vi "test.vi"() -> ()   [LabVIEW 2025]
uses:
  <vilib>/userDefined/High Color/IMAQdx.ctl
  <vilib>/httpClient/POSTBuffer.vi
  <vilib>/vision/driver/NI_Vision_Acquisition_Software.lvlib
  <vilib>/httpClient/LabVIEWHTTPClient.lvlib
  <vilib>/smtpClient/LabVIEWSMTPClient.lvlib
  <vilib>/vision/NI_Vision_Development_Module.lvlib
panel:
  out "Image":T1(plugin-control)
  in  "Salvare imagine":bool
  in  "Pornire achizitie locala imagini":bool
  in  "Stop server":bool
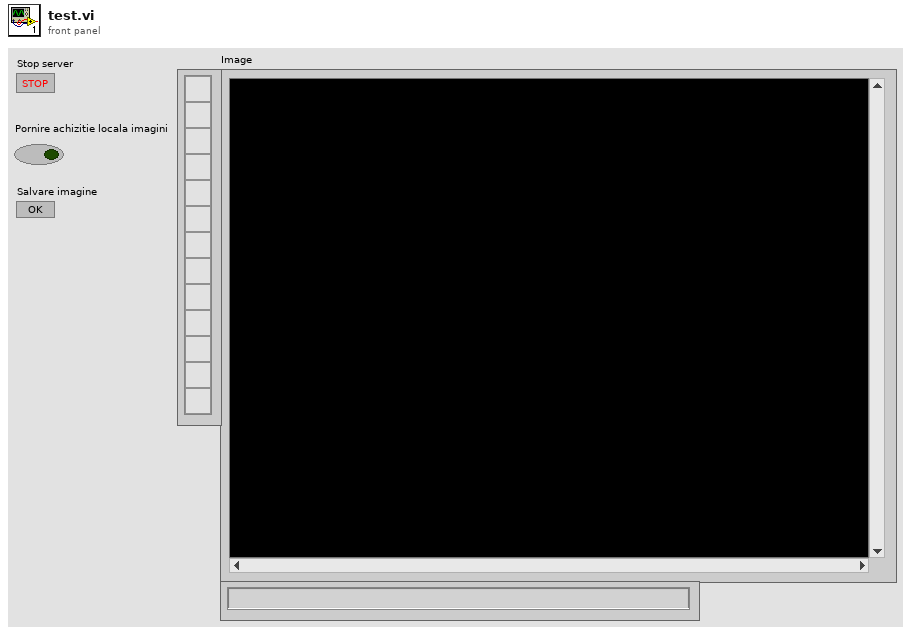
[diagram p1: front panel]
types:
  T1 = typedef "IMAQ Image.ctl" = refnum<image>
  T2 = typedef "Image Type" = u32
  T3 = typedef "IMAQdx.ctl" = refnum<k21>
  T4 = typedef "LabVIEWHTTPClient.lvlib/ClientHandle.ctl" = refnum<k1>
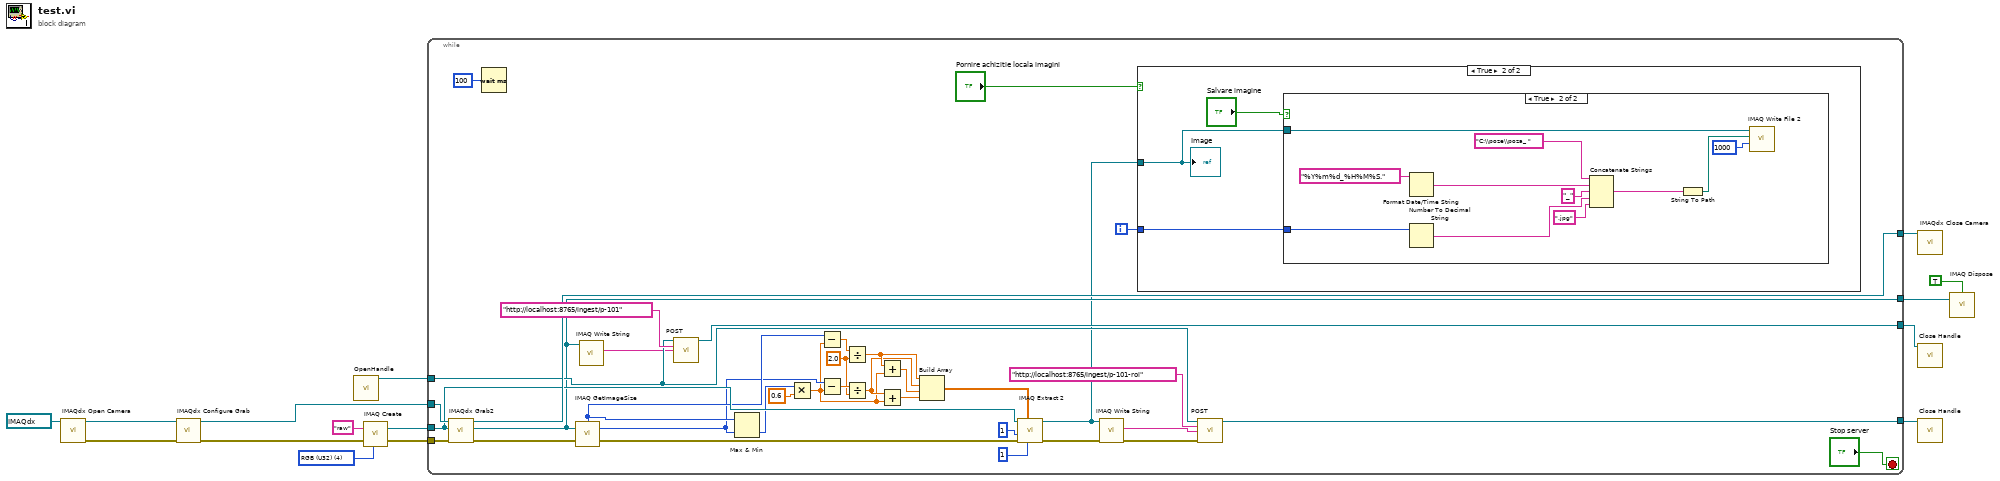
[diagram p0: block diagram]
diagram:
  w3 = T2 4 items=["Grayscale (U8)", "Grayscale (I16)", "Grayscale (SGL)", "Complex (CSG)", "RGB (U32)", "HSL (U32)", "RGB (U64)", "Grayscale (U16)"] ("Image Type")
  n1 = call <vilib>:"IMAQdx Open Camera.vi"("Session In"=T3 "cam1") -> ("error out"=w10:errorcluster, "Session Out"=w13:T3)  [unwired: 9 in]
  n2 = call <vilib>:"IMAQdx Configure Grab.vi"("error in"=w10, "Session In"=w13) -> ("error out"=w9:errorcluster, "Session Out"=w12:T3)  [unwired: 8 in]
  n3 = call <vilib>:"OpenHandle.vi"() -> ("client handle out"=w7:T4)  [unwired: 14 in, 1 out]
  n4 = call "IMAQ Create"("Image Name"="raw", "Image Type"=w3, "error in (no error)"=w9) -> ("New Image"=w14:T1, "error out"=w2:errorcluster)  [unwired: 2 in]
  n5 = while {
    tunnel: w14 -> [w44]
    tunnel: w12 -> [w51]
    tunnel: [w50] -> w11
    tunnel: [w49] -> w8
    tunnel: w7 -> [w45]
    tunnel: [w23] -> w5
    tunnel: w2 -> [w27]
    tunnel: [w30] -> w1
    i -> [w16]
    stop <- "Stop server" stop-if-true
    w37 = 2.0 ("y")
    n6 = call <vilib>:"IMAQdx Grab2.vi"("error in"=w27, "Image In"=w44, "Session In"=w51) -> ("error out"=w26:errorcluster, "Image Out"=w23:T1, "Session Out"=w50:T3)  [unwired: 5 in, 1 out]
    n7 = Wait (ms)(milliseconds to wait=u32 100 ("millisecond timer value")) -> ()  [unwired: 1 out]
    n8 = call "IMAQ GetImageSize"("Image"=w23, "error in (no error)"=w26) -> ("Y Resolution"=w39:i32, "X Resolution"=w43:i32, "error out"=w25:errorcluster)  [unwired: 2 in]
    n9 = call-poly "IMAQ Write String"("Image"=w23) -> ("FileString"=w22:string)  [unwired: 8 in, 2 out]
    n10 = call-poly <vilib>:"POST.vi"("client handle"=w45, "url"="http://localhost:8765/ingest/p-101", "buffer"=w22) -> ("client handle out"=w49:T4)  [unwired: 9 in, 3 out]
    n11 = Max & Min(x=w43, y=w39) -> (min(x,y)=w41:i32)  [unwired: 1 out]
    n12 = Multiply(x=w41, y=0.6) -> (x*y=w33:dbl)
    n13 = Subtract(x=w43, y=w33) -> (x-y=w40:dbl)
    n14 = Subtract(x=w39, y=w33) -> (x-y=w38:dbl)
    n15 = Divide(x=w40, y=w37) -> (x/y=w36:dbl)
    n16 = Divide(x=w38, y=w37) -> (x/y=w34:dbl)
    n17 = Add(x=w36, y=w33) -> (x+y=w35:dbl)
    n18 = Add(x=w34, y=w33) -> (x+y=w32:dbl)
    n19 = Build Array "Build Array"(w36, w34, w35, w32) -> (w31:dbl[])
    n20 = call "IMAQ Extract 2"("Y Step Size"=1, "Optional Rectangle"=w31, "error in (no error)"=w25, "X Step Size"=1, "Image Src"=w44) -> ("error out"=w20:errorcluster, "Image Dst Out"=w17:T1)  [unwired: 5 in]
    n21 = call-poly "IMAQ Write String"("error in (no error)"=w20, "Image"=w17) -> ("error out"=w19:errorcluster, "FileString"=w21:string)  [unwired: 7 in, 1 out]
    n22 = case shown="True" "Pornire achizitie locala imagini" {
      tunnel: w17 -> [_ w52]
      tunnel: w16 -> [_ w53]
      frame False {
      }
      frame True {
        n23 = case shown="True" "Salvare imagine" {
          tunnel: w52 -> [_ w56]
          tunnel: w53 -> [_ w61]
          frame False {
          }
          frame True {
            n24 = Format Date/Time String(time format string (%c)="%Y%m%d_%H%M%S.") -> (date/time string=w63:string)  [unwired: 2 in]
            n25 = Number To Decimal String(number=w61) -> (decimal integer string=w59:string)  [unwired: 1 in]
            n26 = Concatenate Strings "Concatenate Strings"("C:\\poze\\poza_ " ("string"), w63, "_" ("string"), w59, ".jpg" ("string")) -> (w62:string)
            n27 = String To Path(string=w62) -> (path=w57:path)
            n28 = call-poly "IMAQ Write File 2"("Image Quality"=u32 1000, "File Path"=w57, "Image"=w56) -> ()  [unwired: 7 in, 2 out]
          }
        }
        "Image" <- w52
      }
    }
    n29 = call-poly <vilib>:"POST.vi"("client handle"=w45, "url"="http://localhost:8765/ingest/p-101-roi", "buffer"=w21, "error in (no error)"=w19) -> ("client handle out"=w30:T4)  [unwired: 8 in, 3 out]
  }
  n30 = call <vilib>:"IMAQdx Close Camera.vi"("Session In"=w11) -> ()  [unwired: 10 in, 1 out]
  n31 = call <vilib>:"Close Handle.vi"("handle in"=w8) -> ()  [unwired: 13 in, 2 out]
  n32 = call <vilib>:"Close Handle.vi"("handle in"=w1) -> ()  [unwired: 13 in, 2 out]
  n33 = call "IMAQ Dispose"("All Images? (No)"=TRUE, "Image"=w5) -> ()  [unwired: 4 in, 1 out]
